vi "automatic_random.vi"(7 "transition_queue":refnum<queue>, 8 "error in (no error)":errorcluster, 10 "data":variant, 11 "recipe_data":variant) -> (0 "error out":errorcluster)   [LabVIEW 2015, in "example_01.lvlib"]
doc: "automatic_random.vi will generate a random number and communicate it to the recipe_machine via recipe_data."
uses:
  example_01.lvlib
  <userlib>/antonio-alexander/lv-recipe-machine/public/_controls/transition.ctl
  _controls/steps_actions_data.ctl
  _controls/steps_actions.ctl
  <userlib>/antonio-alexander/lv-recipe-machine/lv-recipe-machine.lvlib
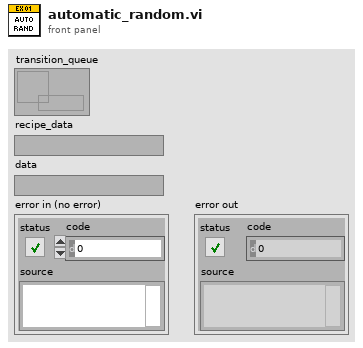
[diagram p1: front panel]
types:
  T1 = typedef "example_01.lvlib/steps_actions.ctl" = enum16{"<steps_actions>", "manual_random", "manual_comparison", "manual_wait", "auto_random", "auto_wait", "criteria_initialize", "criteria_count", "criteria_comparison", "transition_simple", "transition_count", "transition_comparison", "launch_wait", "<null>"}
  T2 = typedef "example_01.lvlib/steps_actions_data.ctl" = cluster{"step_action":T1, "data":variant}
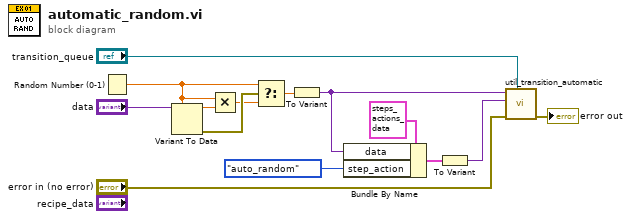
[diagram p0: block diagram]
diagram:
  n1 = Random Number (0-1)() -> (number: 0 to 1=w2:dbl)
  n2 = Variant To Data(type=w2, Variant="data") -> (data=w3:dbl, error out=w14:errorcluster)  [unwired: 1 in]
  n3 = Multiply(x=w2, y=w3) -> (x*y=w4:dbl)
  n4 = Select(t=w2, s=w14, f=w4) -> (s? t:f=w1:dbl)
  n5 = To Variant(anything=w1) -> (Variant=w8:variant)
  n6 = Bundle By Name(cluster=T2 {"step_action"=enum."<steps_actions>", "data"=variant}, "data"=w8, "step_action"=steps_actions."auto_random" ("automatic_steps")) -> (w10:T2)
  n7 = To Variant(anything=w10) -> (Variant=w9:variant)
  n8 = call <userlib>:"util_transition_automatic.vi"("transition_queue"="transition_queue", "error in (no error)"="error in (no error)", "data"=w9, "recipe_data"=w8) -> ("error out"=→"error out":errorcluster)  [unwired: 7 in]
